vi "getTreeSelection.vi"(8 "error in (no error)":errorcluster, 11 "LoggerMonitorControlData":T1) -> (0 "error out":errorcluster, 2 "isDir?":bool, 3 "SelectedPath":string)   [LabVIEW 2015]
uses:
  LoggerMonitorControlData.ctl
  General/RemoteFiles/connectionData.ctl
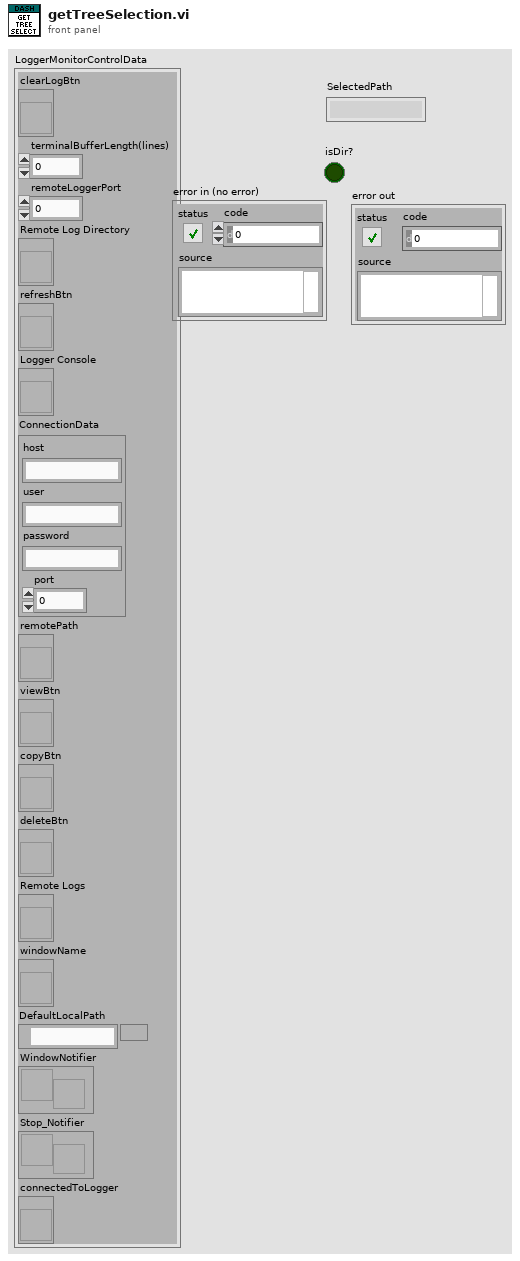
[diagram p1: front panel]
types:
  T1 = typedef "LoggerMonitorControlData.ctl" = cluster{"clearLogBtn":refnum<vi>, "terminalBufferLength(lines)":i32, "remoteLoggerPort":u16, "Remote Log Directory":refnum<vi>, "refreshBtn":refnum<vi>, "Logger Console":refnum<vi>, "ConnectionData":T2, "remotePath":refnum<vi>, "viewBtn":refnum<vi>, "copyBtn":refnum<vi>, "deleteBtn":refnum<vi>, "Remote Logs":refnum<vi>, "windowName":refnum<vi>, "DefaultLocalPath":path, "WindowNotifier":refnum<notifier>, "Stop_Notifier":refnum<notifier>, "connectedToLogger":refnum<vi>}
  T2 = typedef "connectionData.ctl" = cluster{"host":string, "user":string, "password":string, "port":u16}
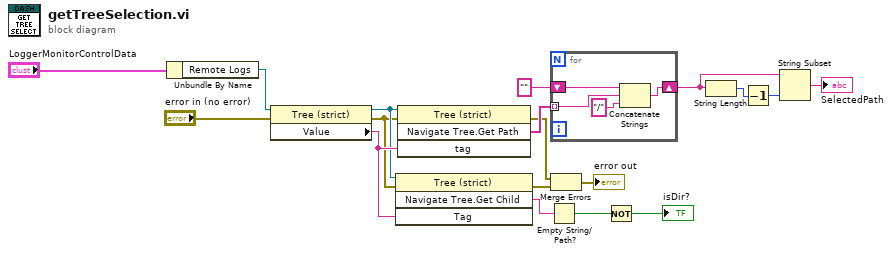
[diagram p0: block diagram]
diagram:
  n1 = Unbundle By Name("LoggerMonitorControlData") -> ("Remote Logs"=w12:refnum<vi>)
  n2 = property class="Tree (strict)"(reference=w12, error in="error in (no error)") -> (reference out=w9:refnum<vi>, error out=w8:errorcluster, "Value"=w10:string)
  n3 = invoke class="Tree (strict)" method="Navigate Tree.Get Child"(reference=w9, error in=w8, "Tag"=w10) -> (error out=w4:errorcluster, "Navigate Tree:Get Child"=w7:string)  [unwired: 1 in, 2 out]
  n4 = invoke class="Tree (strict)" method="Navigate Tree.Get Path"(reference=w9, error in=w8, "tag"=w10) -> (error out=w3:errorcluster, "Navigate Tree:Get Path"=w18:string[])  [unwired: 1 in, 2 out]
  n5 = Empty String/Path?(string/path=w7) -> (empty?=w6:bool)
  n6 = for {
    tunnel: w18 -> [w20] mode=indexing
    shift-right: [w21] -> w14
    shift-left: "" -> [w22]
    n7 = Concatenate Strings(w22, w20, "/" ("string")) -> (w21:string)
  }
  n8 = Merge Errors(w3, w4) -> (→"error out":errorcluster)
  n9 = Not(x=w6) -> (.not. x?=→"isDir?":bool)
  n10 = String Length(string=w14) -> (length=w16:i32)
  n11 = Decrement(x=w16) -> (x-1=w15:i32)
  n12 = String Subset(string=w14, length (rest)=w15) -> (substring=→"SelectedPath":string)  [unwired: 1 in]
